vi "Funnel_Test.vi"(11 "Joystick Controls":T1) -> ()   [LabVIEW 2020]
uses:
  Subsystems/Funnel/Control_States_Funnel.ctl
  Subsystems/Funnel/Funnel_Cluster.ctl
  Globals/Funnel_global.vi
  Utility VIs/Joystick_Controls.ctl
panel:
  in  "funnel_throttle":dbl=1.0
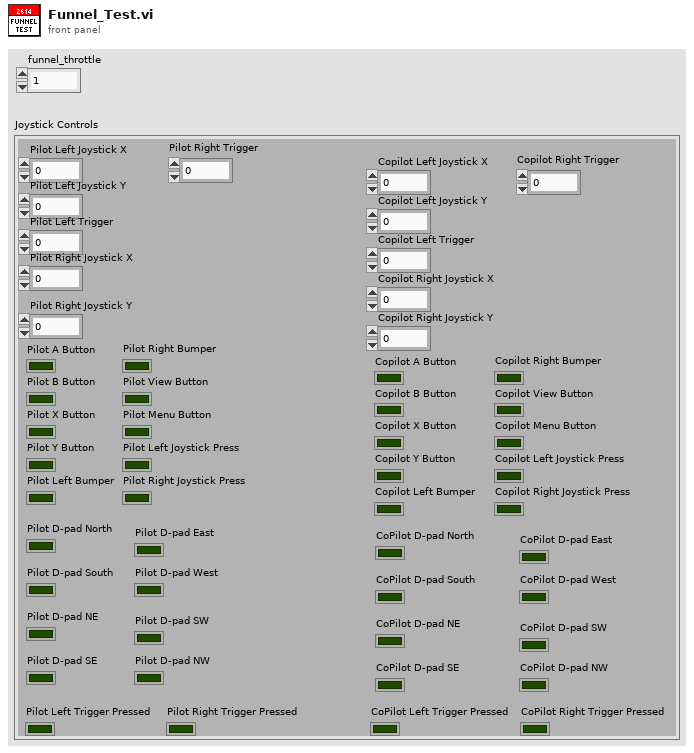
[diagram p1: front panel]
types:
  T1 = typedef "Joystick_Controls.ctl" = cluster{"Pilot Left Joystick X":dbl, "Pilot Left Joystick Y":dbl, "Pilot A Button":bool, "Pilot B Button":bool, "Pilot X Button":bool, "Pilot Y Button":bool, "Pilot Left Bumper":bool, "Pilot Right Bumper":bool, "Pilot View Button":bool, "Pilot Menu Button":bool, "Pilot Left Joystick Press":bool, "Pilot Right Joystick Press":bool, "Pilot Left Trigger":dbl, "Pilot Right Joystick X":dbl, "Pilot Right Joystick Y":dbl, "Pilot Right Trigger":dbl, "Copilot Left Joystick X":dbl, "Copilot Left Joystick Y":dbl, "Copilot A Button":bool, "Copilot B Button":bool, "Copilot X Button":bool, "Copilot Y Button":bool, "Copilot Left Bumper":bool, "Copilot Right Bumper":bool, "Copilot View Button":bool, "Copilot Menu Button":bool, "Copilot Left Joystick Press":bool, "Copilot Right Joystick Press":bool, "Copilot Left Trigger":dbl, "Copilot Right Joystick X":dbl, "Copilot Right Joystick Y":dbl, "Copilot Right Trigger":dbl, "Pilot D-pad North":bool, "Pilot D-pad South":bool, "Pilot D-pad East":bool, "Pilot D-pad West":bool, "Pilot D-pad NE ":bool, "Pilot D-pad SE":bool, "Pilot D-pad SW":bool, "Pilot D-pad NW":bool, "CoPilot D-pad North":bool, "CoPilot D-pad South":bool, "CoPilot D-pad East":bool, "CoPilot D-pad West":bool, "CoPilot D-pad NE":bool, "CoPilot D-pad SE":bool, "CoPilot D-pad SW":bool, "CoPilot D-pad NW":bool, "Pilot Left Trigger Pressed":bool, "Pilot Right Trigger Pressed":bool, "CoPilot Left Trigger Pressed":bool, "CoPilot Right Trigger Pressed":bool}
  T2 = typedef "Funnel_Cluster.ctl" = cluster{"Control States":T3, "%Vbus":dbl}
  T3 = typedef "Control_States_Funnel.ctl" = enum16{"No_Op", "Manual_Op", "Load", "Firing", "Outtake"}
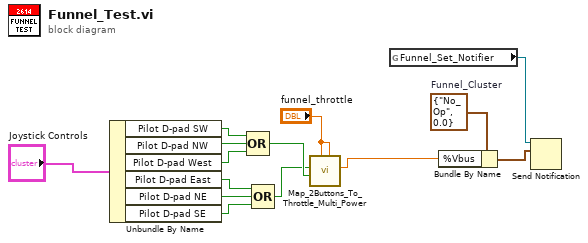
[diagram p0: block diagram]
diagram:
  w13 = T2 {"Control States"=enum."No_Op", "%Vbus"=0.0}  # Funnel_Cluster
  n1 = Unbundle By Name("Joystick Controls") -> ("Pilot D-pad SW"=w10:bool, "Pilot D-pad NW"=w9:bool, "Pilot D-pad West"=w8:bool, "Pilot D-pad East"=w7:bool, "Pilot D-pad NE"=w6:bool, "Pilot D-pad SE"=w5:bool)
  n2 = Compound Arithmetic op=OR(w10, w9, w8) -> (w4:bool)
  n3 = Compound Arithmetic op=OR(w7, w6, w5) -> (w3:bool)
  n4 = call "Map_2Buttons_To_Throttle_Multi_Power.vi"("Power_Down"="funnel_throttle", "Power_Up"="funnel_throttle", "Down"=w4, "Up"=w3) -> ("Throttle"=w1:dbl)  [unwired: 7 in]
  n5 = global read "Funnel_global.vi" "Funnel_Set_Notifier"() -> (w11:refnum<notifier>)
  n6 = Bundle By Name(cluster=w13, "%Vbus"=w1) -> (w12:T2)
  n7 = Send Notification(notification=w12, notifier=w11) -> ()  [unwired: 1 in, 2 out]
